vi "connectPubDataSubscribe.vi"(8 "error in (no error)":errorcluster, 11 "MiddlewareSALThisComponent in":refnum<class "MiddlewareSALThisComponent.lvclass">) -> (0 "error out":errorcluster, 3 "MiddlewareSALThisComponent out":refnum<class "MiddlewareSALThisComponent.lvclass">)   [LabVIEW 2016, in "MiddlewareSALThisComponent.lvclass"]
uses:
  MiddlewareSALThisComponent.lvclass
  ts_sallv_exa/SALLV_EXA.lvlib
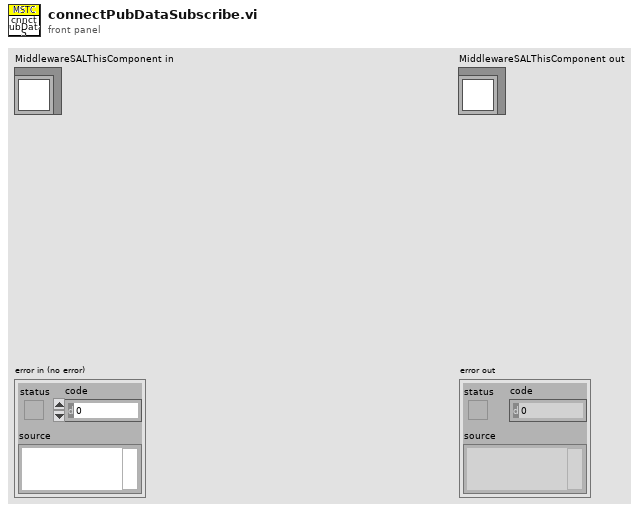
[diagram p1: front panel]
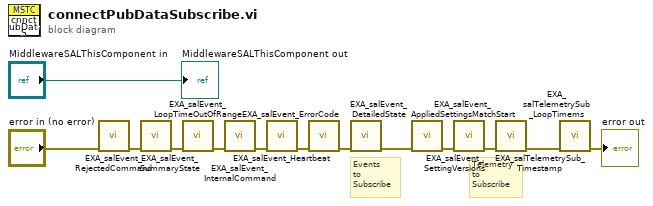
[diagram p0: block diagram]
diagram:
  # "Telemetry \nto \nSubscribe"
  # "Events \nto \nSubscribe"
  n1 = call "EXA_salEvent_RejectedCommand.vi"("error in (no error)"="error in (no error)") -> ("error out"=w10:errorcluster)  [unwired: 9 in, 1 out]
  n2 = call "EXA_salEvent_SummaryState.vi"("error in (no error)"=w10) -> ("error out"=w9:errorcluster)  [unwired: 9 in, 1 out]
  n3 = call "EXA_salEvent_LoopTimeOutOfRange.vi"("error in (no error)"=w9) -> ("error out"=w8:errorcluster)  [unwired: 9 in, 1 out]
  n4 = call "EXA_salEvent_InternalCommand.vi"("error in (no error)"=w8) -> ("error out"=w2:errorcluster)  [unwired: 9 in, 1 out]
  n5 = call "EXA_salEvent_Heartbeat.vi"("error in (no error)"=w2) -> ("error out"=w7:errorcluster)  [unwired: 9 in, 1 out]
  n6 = call "EXA_salEvent_ErrorCode.vi"("error in (no error)"=w7) -> ("error out"=w6:errorcluster)  [unwired: 9 in, 1 out]
  n7 = call "EXA_salEvent_DetailedState.vi"("error in (no error)"=w6) -> ("error out"=w1:errorcluster)  [unwired: 9 in, 1 out]
  n8 = call "EXA_salEvent_AppliedSettingsMatchStart.vi"("error in (no error)"=w1) -> ("error out"=w5:errorcluster)  [unwired: 9 in, 1 out]
  n9 = call "EXA_salEvent_SettingVersions.vi"("error in (no error)"=w5) -> ("error out"=w3:errorcluster)  [unwired: 9 in, 1 out]
  n10 = call "EXA_salTelemetrySub_Timestamp.vi"("error in (no error)"=w3) -> ("error out"=w11:errorcluster)  [unwired: 9 in, 1 out]
  n11 = call "EXA_salTelemetrySub_LoopTimems.vi"("error in (no error)"=w11) -> ("error out"=→"error out":errorcluster)  [unwired: 9 in, 1 out]
  "MiddlewareSALThisComponent out" <- "MiddlewareSALThisComponent in"
